vi "CRYPlot Table.vi"(6 "Result Rows In":i32[](array[numeric]), 7 "pGraph VI In":refnum<vi>, 8 "Graph Set?":bool, 9 "Flattened Property":string, 10 "Value Rows In":i32[](array[numeric]), 11 "Curve Rows In":i32[](array[numeric])) -> (0 "Value Name":string[](array[string]), 1 "Value Rows Out":i32[](array[numeric]), 2 "Curve Name":string[](array[string]), 3 "Curve Rows Out":i32[](array[numeric]), 4 "Result Rows Out":i32[](array[numeric]), 5 "Result Name":string[](array[string]))   [LabVIEW 2013]
uses:
  CRYWindow/DataView/Control/CRYTable Property.ctl
panel:
  in  "Table Property":T1 {"Precision" items=["Digits of precision", "Significant digits"]}
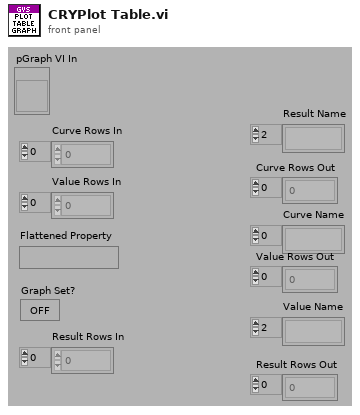
[diagram p1: front panel]
types:
  T1 = typedef "CRYTable Property.ctl" = cluster{"Reset All Columns":bool, "Transpose":bool, "Display Units":bool, "Notation":u16, "Digits":u16, "Precision":u16, "Hide Traling Zeros":bool, "Column Width":u16, "Row Header Width":u16, "Show vertical scroll bar":bool, "Show horizontal scroll bar":bool}
  T2 = typedef "CRYData Cluster.ctl" = cluster{"Name":string, "Curve":cluster{"x":dbl, "y":dbl, "z":dbl}[], "X data":u16, "Y data":u16, "Z data":u16, "X axis":u16, "Y axis":u16, "Z axis":u16, "X unit":string, "Y unit":string, "Z unit":string, "X dB ref":dbl, "Y dB ref":dbl, "Z dB ref":dbl, "single val":bool, "protected":bool, "display X":bool, "display Y":bool, "display Z":bool, "Test Info":string, "Step No.":i32, "Plot Settings":cluster{"Color":u32, "Interpolation":u8, "Point Style":u8, "Line Style":u8, "Point Color":u32, "Line Width":u8, "Bar Plot Style":u8, "Fill To":i16}, "AutoProtect":bool}
  T3 = typedef "CRYResult Cluster.ctl" = cluster{"Name":string, "Margin":dbl, "unit":string, "Verdict":bool, "Limit":string, "Max/Min":string, "protected":bool, "Step No.":i32, "Test Info":string, "AutoProtect":bool}
  T4 = cluster{"left":i16, "top":i16, "right":i16, "bottom":i16}
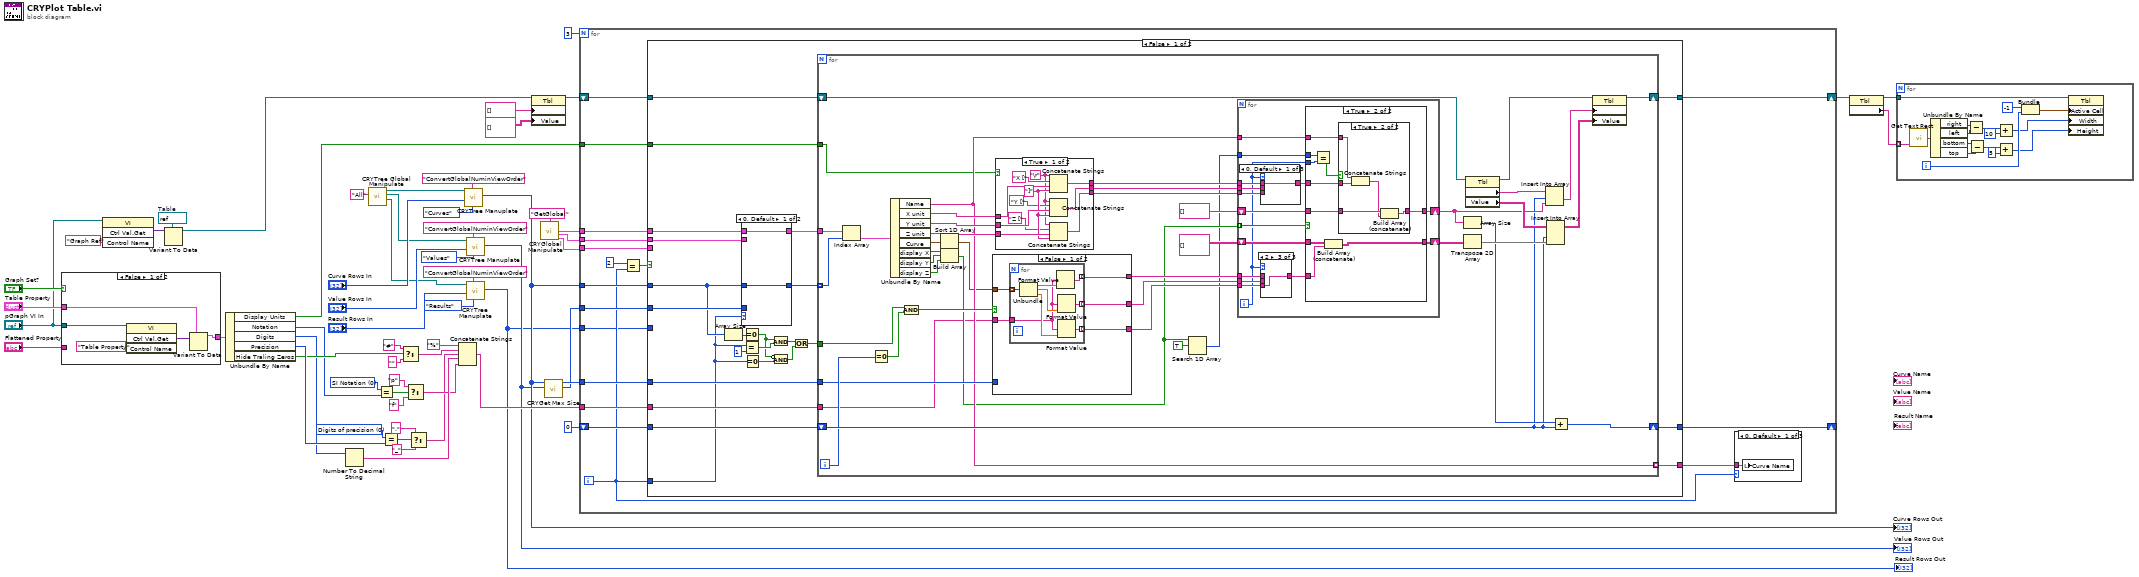
[diagram p0: block diagram]
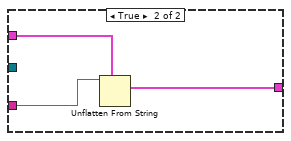
[diagram p2: hidden frame]
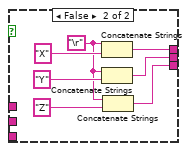
[diagram p4: hidden frame]
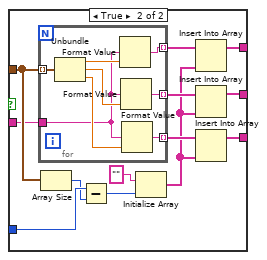
[diagram p5: hidden frame]
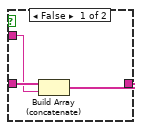
[diagram p11: hidden frame]
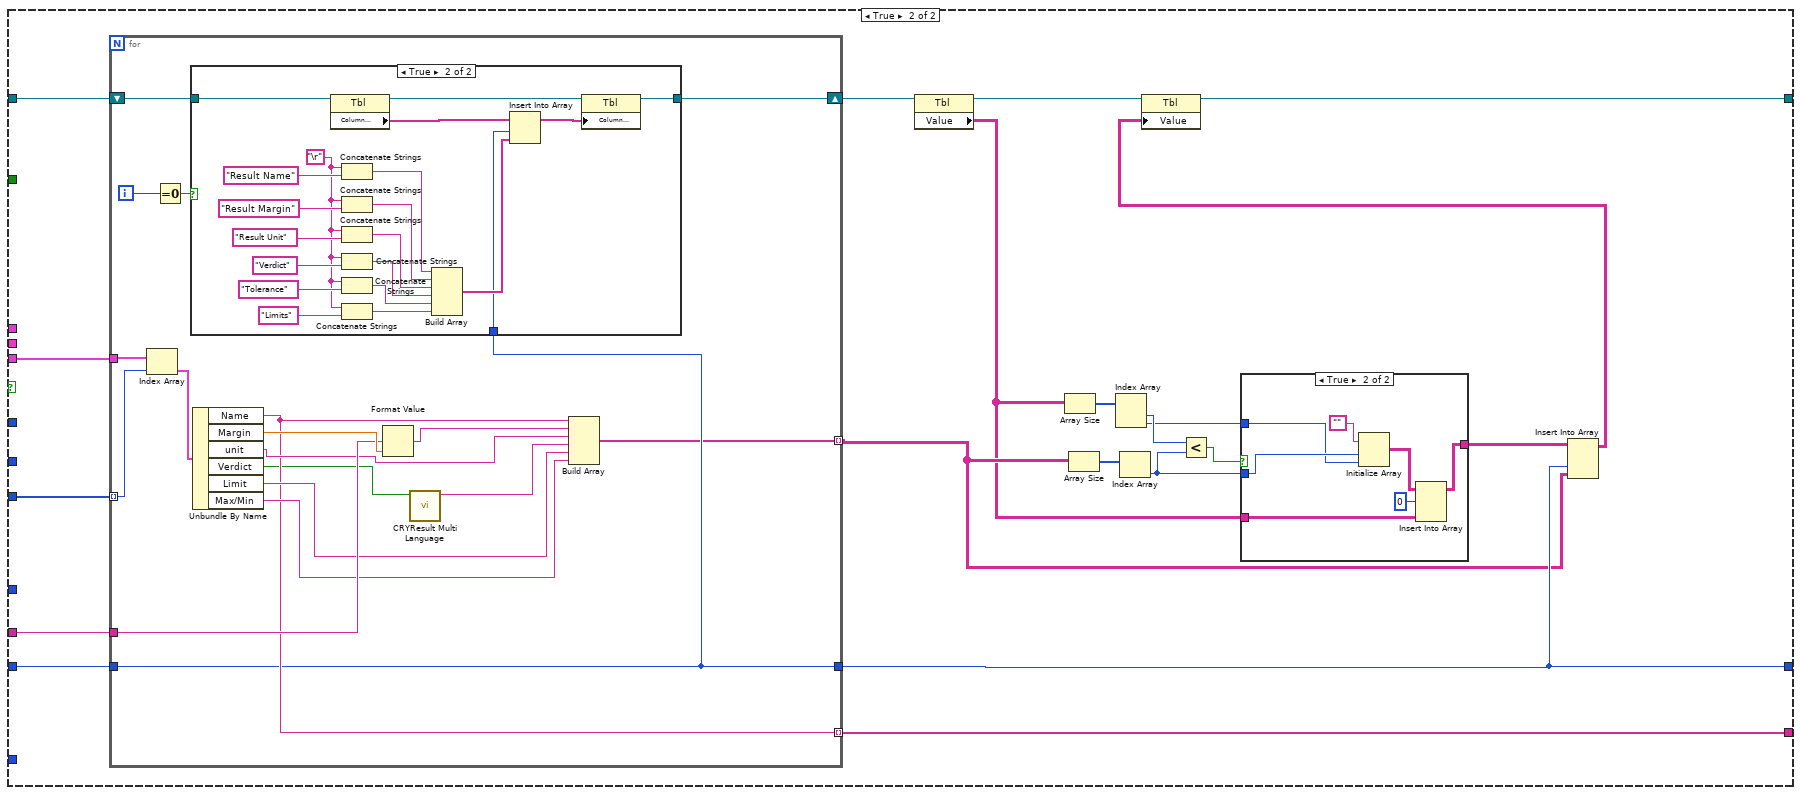
[diagram p12: hidden frame]
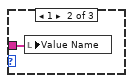
[diagram p15: hidden frame]
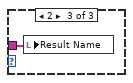
[diagram p16: hidden frame]
diagram:
  w23 = refnum<vi> refnum  # Table
  w40 = u16 0 items=["Digits of precision", "Significant digits"] ("Precision")
  w39 = u16 0 items=["SI Notation", "Floating point"] ("Notation")
  n1 = case shown="False" "Graph Set?" {
    tunnel: "Table Property" -> [w62 w67]
    tunnel: [w61 w65] -> w32
    tunnel: "pGraph VI In" -> [w60 _]
    tunnel: "Flattened Property" -> [_ w66]
    frame False {
      n2 = invoke class="VI" method="Ctrl Val.Get"(reference=w60, "Control Name"="Table Property") -> ("Get Control Value Variant"=w63:variant)  [unwired: 2 in, 3 out]
      n3 = Variant To Data(type=w62, Variant=w63) -> (data=w61:T1)  [unwired: 1 in, 1 out]
    }
    frame True {
      n4 = Unflatten From String(type=w67, binary string=w66) -> (value=w65:T1)  [unwired: 3 in, 2 out]
    }
  }
  n5 = invoke class="VI" method="Ctrl Val.Get"(reference="pGraph VI In", "Control Name"="Graph Ref") -> ("Get Control Value Variant"=w22:variant)  [unwired: 2 in, 3 out]
  n6 = Variant To Data(type=w23, Variant=w22) -> (data=w21:refnum<vi>)  [unwired: 1 in, 1 out]
  n7 = Unbundle By Name(w32) -> ("Display Units"=w29:bool, "Notation"=w36:u16, "Digits"=w35:u16, "Precision"=w38:u16, "Hide Traling Zeros"=w37:bool)
  n8 = Number To Decimal String(number=w35) -> (decimal integer string=w53:string)  [unwired: 1 in]
  n9 = call "CRYTree Global Manipulate.vi"("sOption"="All") -> ("Results Tree"=w4:refnum<vi>, "Values Tree"=w5:refnum<vi>, "Tree/Curve Tree"=w6:refnum<vi>)  [unwired: 7 in, 1 out]
  n10 = Equal?(x=w39, y=w36) -> (x = y?=w42:bool)
  n11 = Equal?(x=w40, y=w38) -> (x = y?=w48:bool)
  n12 = Select(t="#" ("format string"), s=w37, f="" ("format string")) -> (s? t:f=w47:string)
  n13 = Select(t="p" ("string"), s=w42, f="f" ("string")) -> (s? t:f=w52:string)
  n14 = Select(t=".", s=w48, f="_") -> (s? t:f=w49:string)
  n15 = Concatenate Strings("%" ("string"), w47, w49, w53, w52) -> (w34:string)
  n16 = call "CRYTree Manuplate.vi"("Type"=enum16{"Curves", "Values", "Results", "WFM"}."Curves", "sAction"="ConvertGlobalNuminViewOrder", "nData"="Curve Rows In", "Tree in"=w6) -> ("nData Out"=w13:i32[])  [unwired: 4 in, 3 out]
  "Curve Rows Out" <- w13
  n17 = call "CRYTree Manuplate.vi"("Type"=enum16{"Curves", "Values", "Results", "WFM"}."Values", "sAction"="ConvertGlobalNuminViewOrder", "nData"="Value Rows In", "Tree in"=w5) -> ("nData Out"=w10:i32[])  [unwired: 4 in, 3 out]
  "Value Rows Out" <- w10
  n18 = call "CRYTree Manuplate.vi"("Type"=enum16{"Curves", "Values", "Results", "WFM"}."Results", "sAction"="ConvertGlobalNuminViewOrder", "nData"="Result Rows In", "Tree in"=w4) -> ("nData Out"=w8:i32[])  [unwired: 4 in, 3 out]
  "Result Rows Out" <- w8
  n19 = property class="Tbl"(reference=w21, "Column Headers[]"=string[] [] ("Column Header Strings[]"), "Value"=string[][] [] ("Item Names")) -> (reference out=w59:refnum<vi>)  [unwired: 1 in, 1 out]
  n20 = call "CRYGlobal Manipulate.vi"("sAction"="GetGlobal") -> ("Curves Out"=w18:T2[], "Values Out"=w17:T2[], "Results Out"=w19:T3[])  [unwired: 8 in, 4 out]
  n21 = call "CRYGet Max Size.vi"("Value Rows"=w10, "Curve Rows"=w13) -> ("Max Size"=w54:i32)  [unwired: 9 out]
  n22 = for {
    N: 3 -> [_]
    tunnel: w18 -> [w84]
    tunnel: w13 -> [w78]
    tunnel: w17 -> [w83]
    tunnel: w10 -> [w82]
    shift-right: [w79] -> _
    shift-left: 0 -> [w80]
    tunnel: w54 -> [w77]
    tunnel: w34 -> [w76]
    tunnel: w29 -> [w75]
    tunnel: w19 -> [w69]
    shift-right: [w73] -> w28
    shift-left: w59 -> [w74]
    tunnel: w8 -> [w68]
    i -> [w71]
    n23 = Equal?(x=2, y=w71) -> (x = y?=w72:bool)
    n24 = case shown="False" w72 {
      tunnel: w84 -> [w106 _]
      tunnel: w83 -> [w104 _]
      tunnel: w82 -> [w103 _]
      tunnel: [w102 w265] -> w81
      tunnel: w80 -> [w101 w263]
      tunnel: [w100 w254] -> w79
      tunnel: w78 -> [w99 _]
      tunnel: w71 -> [w85 _]
      tunnel: w77 -> [w90 _]
      tunnel: w76 -> [w89 w266]
      tunnel: w75 -> [w88 _]
      tunnel: w74 -> [w87 w264]
      tunnel: [w86 w260] -> w73
      tunnel: w69 -> [_ w268]
      tunnel: w68 -> [_ w267]
      frame False {
        n25 = Array Size(array=w99) -> (size(s)=w98:i32)
        n26 = case shown="0, Default" w85 {
          tunnel: [w109 w110] -> w107
          tunnel: w99 -> [w109 _]
          tunnel: [w108 w111] -> w105
          tunnel: w106 -> [w108 _]
          tunnel: w104 -> [_ w111]
          tunnel: w103 -> [_ w110]
          frame 0, Default {
          }
          frame 1 {
          }
        }
        n27 = Equal To 0?(x=w98) -> (x = 0?=w95:bool)
        n28 = Equal?(x=w85, y=1) -> (x = y?=w96:bool)
        n29 = Equal To 0?(x=w85) -> (x = 0?=w94:bool)
        n30 = And(x=w95, y=w96) -> (x .and. y?=w93:bool)
        n31 = Compound Arithmetic op=AND(invert w95, w94) -> (w92:bool)
        n32 = Or(x=w93, y=w92) -> (x .or. y?=w91:bool)
        n33 = for {
          tunnel: w105 -> [w154]
          tunnel: w107 -> [w151] mode=indexing
          tunnel: [w119] -> w102 mode=indexing
          shift-right: [w129] -> w100
          shift-left: w101 -> [w127]
          tunnel: w91 -> [w122]
          tunnel: w90 -> [w120]
          tunnel: w89 -> [w115]
          tunnel: w88 -> [w114]
          shift-right: [w113] -> w86
          shift-left: w87 -> [w145]
          i -> [w126]
          n34 = Index Array(array=w154, index=w151) -> (element=w121:T2)
          n35 = Equal To 0?(x=w126) -> (x = 0?=w124:bool)
          n36 = Unbundle By Name(w121) -> ("Name"=w119:string, "X unit"=w152:string, "Y unit"=w153:string, "Z unit"=w144:string, "Curve"=w125:cluster{"x":dbl, "y":dbl, "z":dbl}[], "display X"=w137:bool, "display Y"=w139:bool, "display Z"=w138:bool)
          n37 = Compound Arithmetic op=AND(w122, w124) -> (w123:bool)
          n38 = Sort 1D Array(array=w125) -> (sorted array=w112:cluster{"x":dbl, "y":dbl, "z":dbl}[])
          n39 = Build Array(w137, w139, w138) -> (w118:bool[])
          n40 = case shown="False" w123 {
            tunnel: [w177 w192] -> w148
            tunnel: [w176 w191] -> w147
            tunnel: [w175 w190] -> w142
            tunnel: w112 -> [w174 w198]
            tunnel: w120 -> [_ w197]
            tunnel: w115 -> [w173 w186]
            frame False {
              n41 = for {
                tunnel: w174 -> [w185] mode=indexing
                tunnel: [w184] -> w177 mode=indexing
                tunnel: [w183] -> w176 mode=indexing
                tunnel: [w182] -> w175 mode=indexing
                tunnel: w173 -> [w178]
                n42 = Unbundle(w185) -> ("x"=w179:dbl, "y"=w180:dbl, "z"=w181:dbl)
                n43 = Format Value(format string=w178, value (0)=w179) -> (output string=w184:string)  [unwired: 1 in]
                n44 = Format Value(format string=w178, value (0)=w180) -> (output string=w183:string)  [unwired: 1 in]
                n45 = Format Value(format string=w178, value (0)=w181) -> (output string=w182:string)  [unwired: 1 in]
              }
            }
            frame True {
              n46 = for {
                tunnel: w198 -> [w206] mode=indexing
                tunnel: [w205] -> w193 mode=indexing
                tunnel: [w204] -> w189 mode=indexing
                tunnel: [w203] -> w188 mode=indexing
                tunnel: w186 -> [w199]
                n47 = Unbundle(w206) -> ("x"=w200:dbl, "y"=w201:dbl, "z"=w202:dbl)
                n48 = Format Value(format string=w199, value (0)=w200) -> (output string=w205:string)  [unwired: 1 in]
                n49 = Format Value(format string=w199, value (0)=w201) -> (output string=w204:string)  [unwired: 1 in]
                n50 = Format Value(format string=w199, value (0)=w202) -> (output string=w203:string)  [unwired: 1 in]
              }
              n51 = Array Size(array=w198) -> (size(s)=w196:i32)
              n52 = Subtract(x=w197, y=w196) -> (x-y=w194:i32)
              n53 = Initialize Array("", w194) -> (w187:string[])
              n54 = Insert Into Array(array=w193, new element=w187) -> (w192:string[])  [unwired: 1 in]
              n55 = Insert Into Array(array=w189, new element=w187) -> (w191:string[])  [unwired: 1 in]
              n56 = Insert Into Array(array=w188, new element=w187) -> (w190:string[])  [unwired: 1 in]
            }
          }
          n57 = case shown="True" w114 {
            tunnel: w153 -> [w164 _]
            tunnel: w152 -> [w163 _]
            tunnel: [w162 w171] -> w150
            tunnel: [w161 w170] -> w149
            tunnel: w144 -> [w160 _]
            tunnel: [w158 w169] -> w143
            frame True {
              w155 = "\r"
              w159 = "]" ("string")
              n58 = Concatenate Strings(w155, "X [", w163, w159) -> (w162:string)
              n59 = Concatenate Strings(w155, "Y [", w164, w159) -> (w161:string)
              n60 = Concatenate Strings(w155, "Z [", w160, w159) -> (w158:string)
            }
            frame False {
              w166 = "\r"
              n61 = Concatenate Strings(w166, "X") -> (w171:string)
              n62 = Concatenate Strings(w166, "Y") -> (w170:string)
              n63 = Concatenate Strings(w166, "Z") -> (w169:string)
            }
          }
          n64 = Search 1D Array(1D array=w118, element=TRUE) -> (index of element=w116:i32)  [unwired: 1 out]
          n65 = for {
            tunnel: w150 -> [w221]
            tunnel: w149 -> [w220]
            tunnel: w148 -> [w218]
            tunnel: w147 -> [w217]
            tunnel: w143 -> [w219]
            tunnel: w142 -> [w216]
            tunnel: w118 -> [w222] mode=indexing
            shift-right: [w212] -> w132
            shift-left: string[] [] -> [w210]
            shift-right: [w211] -> w134
            shift-left: string[][] [] -> [w213]
            tunnel: w119 -> [w209]
            tunnel: w116 -> [w207]
            i -> [w208]
            n66 = case shown="0, Default" w208 {
              tunnel: w221 -> [w226 _ _]
              tunnel: [w226 w227 w228] -> w215
              tunnel: w220 -> [_ w227 _]
              tunnel: w219 -> [_ _ w228]
              frame 0, Default {
              }
              frame 1 {
              }
              frame 2 {
              }
            }
            n67 = case shown="2" w208 {
              tunnel: w218 -> [w223 _ _]
              tunnel: w217 -> [_ w224 _]
              tunnel: w216 -> [_ _ w225]
              tunnel: [w223 w224 w225] -> w214
              frame 0, Default {
              }
              frame 1 {
              }
              frame 2 {
              }
            }
            n68 = case shown="True" w222 {
              tunnel: [w229 w240] -> w211
              tunnel: w215 -> [_ w235]
              tunnel: w214 -> [_ w238]
              tunnel: w210 -> [w230 w237]
              tunnel: w213 -> [w229 w239]
              tunnel: [w230 w236] -> w212
              tunnel: w209 -> [_ w234]
              tunnel: w208 -> [_ w233]
              tunnel: w207 -> [_ w232]
              frame False {
              }
              frame True {
                n69 = Equal?(x=w232, y=w233) -> (x = y?=w231:bool)
                n70 = Build Array (concatenate)(w239, w238) -> (w240:string[][])
                n71 = case shown="True" w231 {
                  tunnel: w237 -> [w243 w248]
                  tunnel: [w242 w247] -> w236
                  tunnel: w235 -> [w241 w245]
                  tunnel: w234 -> [_ w246]
                  frame False {
                    n72 = Build Array (concatenate)(w243, w241) -> (w242:string[])
                  }
                  frame True {
                    n73 = Concatenate Strings(w246, w245) -> (w244:string)
                    n74 = Build Array (concatenate)(w248, w244) -> (w247:string[])
                  }
                }
              }
            }
          }
          n75 = Array Size(array=w132) -> (size(s)=w130:i32)
          n76 = Transpose 2D Array(2D array=w134) -> (transposed array=w135:string[][])
          n77 = property class="Tbl"(reference=w145) -> (reference out=w128:refnum<vi>, "Column Headers[]"=w141:string[], "Value"=w140:string[][])  [unwired: 1 in, 1 out]
          n78 = Insert Into Array(array=w141, index=w127, new element=w132) -> (w131:string[])
          n79 = Insert Into Array(array=w140, index (col)=w127, new element=w135) -> (w146:string[][])  [unwired: 1 in]
          n80 = Add(x=w130, y=w127) -> (x+y=w129:i32)
          n81 = property class="Tbl"(reference=w128, "Column Headers[]"=w131, "Value"=w146) -> (reference out=w113:refnum<vi>)  [unwired: 1 in, 1 out]
        }
      }
      frame True {
        n82 = for {
          tunnel: w268 -> [w294]
          tunnel: w267 -> [w293] mode=indexing
          tunnel: w266 -> [w290]
          tunnel: [w285] -> w265 mode=indexing
          shift-right: [w280] -> w261
          shift-left: w264 -> [w284]
          tunnel: w263 -> [w283]
          tunnel: [w283] -> w254
          tunnel: [w279] -> w253 mode=indexing
          i -> [w281]
          n83 = Index Array(array=w294, index=w293) -> (element=w292:T3)
          n84 = Equal To 0?(x=w281) -> (x = 0?=w282:bool)
          n85 = case shown="True" w282 {
            tunnel: w284 -> [w295 w311]
            tunnel: w283 -> [_ w297]
            tunnel: [w295 w296] -> w280
            frame False {
            }
            frame True {
              w304 = "\r"
              n86 = property class="Tbl"(reference=w311) -> (reference out=w315:refnum<vi>, "Column Headers[]"=w312:string[])  [unwired: 1 in, 1 out]
              n87 = Concatenate Strings(w304, "Result Name") -> (w310:string)
              n88 = Concatenate Strings(w304, "Result Margin") -> (w298:string)
              n89 = Concatenate Strings(w304, "Result Unit") -> (w299:string)
              n90 = Concatenate Strings(w304, "Verdict") -> (w300:string)
              n91 = Concatenate Strings(w304, "Tolerance") -> (w301:string)
              n92 = Concatenate Strings(w304, "Limits") -> (w302:string)
              n93 = Build Array(w310, w298, w299, w300, w301, w302) -> (w314:string[])
              n94 = Insert Into Array(array=w312, index=w297, new element=w314) -> (w313:string[])
              n95 = property class="Tbl"(reference=w315, "Column Headers[]"=w313) -> (reference out=w296:refnum<vi>)  [unwired: 1 in, 1 out]
            }
          }
          n96 = Unbundle By Name(w292) -> ("Name"=w285:string, "Margin"=w291:dbl, "unit"=w288:string, "Verdict"=w278:bool, "Limit"=w287:string, "Max/Min"=w286:string)
          n97 = Format Value(format string=w290, value (0)=w291) -> (output string=w289:string)  [unwired: 1 in]
          n98 = call "CRYResult Multi Language.vi"("Verdict"=w278) -> ("ASCII out"=w277:string)  [unwired: 10 in]
          n99 = Build Array(w285, w289, w288, w277, w287, w286) -> (w279:string[])
        }
        n100 = property class="Tbl"(reference=w261) -> (reference out=w262:refnum<vi>, "Value"=w252:string[][])  [unwired: 1 in, 1 out]
        n101 = Array Size(array=w252) -> (size(s)=w259:i32[])
        n102 = Array Size(array=w253) -> (size(s)=w256:i32[])
        n103 = Index Array(array=w259) -> (element #1=w258:i32, element #2=w249:i32)  [unwired: 2 in]
        n104 = Index Array(array=w256) -> (element=w255:i32)  [unwired: 1 in]
        n105 = Less?(x=w258, y=w255) -> (x < y?=w257:bool)
        n106 = case shown="True" w257 {
          tunnel: w255 -> [_ w275]
          tunnel: w252 -> [w269 w273]
          tunnel: [w269 w272] -> w251
          tunnel: w249 -> [_ w271]
          frame False {
          }
          frame True {
            n107 = Initialize Array("", w275, w271) -> (w274:string[][])
            n108 = Insert Into Array(array=w274, index (row)=0, new element=w273) -> (w272:string[][])  [unwired: 1 in]
          }
        }
        n109 = Insert Into Array(array=w251, index (col)=w254, new element=w253) -> (w250:string[][])  [unwired: 1 in]
        n110 = property class="Tbl"(reference=w262, "Value"=w250) -> (reference out=w260:refnum<vi>)  [unwired: 1 in, 1 out]
      }
    }
    n111 = case shown="0, Default" w71 {
      tunnel: w81 -> [w316 w317 w318]
      frame 0, Default {
        n112 = local write "Curve Name"(w316) -> ()
      }
      frame 1 {
        n113 = local write "Value Name"(w317) -> ()
      }
      frame 2 {
        n114 = local write "Result Name"(w318) -> ()
      }
    }
  }
  n115 = property class="Tbl"(reference=w28) -> (reference out=w27:refnum<vi>, "Column Headers[]"=w26:string[])  [unwired: 1 in, 1 out]
  n116 = for {
    tunnel: w27 -> [w320]
    tunnel: w26 -> [w319] mode=indexing
    i -> [w334]
    n117 = call <vilib>:"Get Text Rect.vi"("text"=w319) -> ("rect"=w329:T4)  [unwired: 5 in, 3 out]
    n118 = Unbundle By Name(w329) -> ("right"=w327:i16, "left"=w328:i16, "bottom"=w325:i16, "top"=w324:i16)
    n119 = Subtract(x=w327, y=w328) -> (x-y=w326:i16)
    n120 = Subtract(x=w325, y=w324) -> (x-y=w322:i16)
    n121 = Add(x=w326, y=i16 10) -> (x+y=w330:i16)
    n122 = Add(x=w322, y=i16 5) -> (x+y=w321:i16)
    n123 = Bundle("Numeric"=i16 -1, w334) -> (w331:cluster{"Numeric":i16, i32})  [unwired: 1 out]
    n124 = property class="Tbl"(reference=w320, "Active Cell"=w331, "Width"=w330, "Height"=w321) -> ()  [unwired: 1 in, 2 out]
  }
